vi "ExSpectGetMirrorInfo.vi"() -> ()   [LabVIEW 2010]
panel:
  out "Position":string
  in  "Mirror Number":i16=1 min=1 max=2 step=1
  out "error out":errorcluster
  in  "error in (no error)":errorcluster
  # "ExSpectGetMirrorInfo.vi\n(Normal Spectrograph via USB/COM port)\nThis VI will read the current position of the selected mirror."
  # "1 = Entrance\n 2 = Exit"
  # "NOTES:\nA properly configured spectometer .ini must be present in the LabVIEW folder for spectrograph operation.\n\nConsult the Toolkit documentation for more information on how to configure this file."
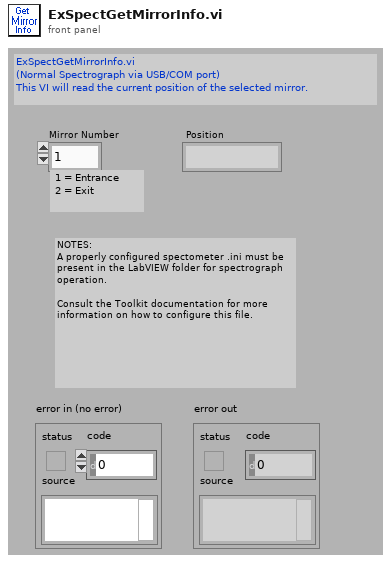
[diagram p1: front panel]
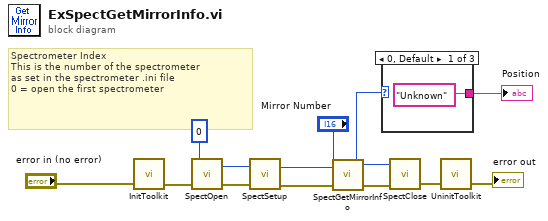
[diagram p0: block diagram]
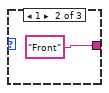
[diagram p2: hidden frame]
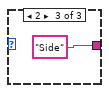
[diagram p3: hidden frame]
diagram:
  # "Spectrometer Index\nThis is the number of the spectrometer\nas set in the spectrometer .ini file\n0 = open the first spectrometer"
  n1 = call <userlib>:"InitToolkit.vi"("error in"="error in (no error)") -> ("error out"=w13:errorcluster)
  n2 = call <userlib>:"SpectOpen.vi"("error in"=w13, "Spectrometer ID"=0) -> ("error out"=w12:errorcluster, "Spectrometer Handle"=w8:u32)  [unwired: 1 in]
  n3 = call <userlib>:"SpectSetup.vi"("error in"=w12, "Spectrometer Handle"=w8) -> ("error out"=w7:errorcluster, "Spectrometer Handle"=w5:u32)
  n4 = call <userlib>:"SpectGetMirrorInfo.vi"("error in"=w7, "Mirror"="Mirror Number", "Spectrometer Handle"=w5) -> ("error out"=w6:errorcluster, "Position"=w2:i16, "Spectrometer Handle"=w3:u32)
  n5 = case shown="0, Default" w2 {
    tunnel: ["Unknown" "Front" "Side"] -> w1
    frame 0, Default {
    }
    frame 1 {
    }
    frame 2 {
    }
  }
  "Position" <- w1
  n6 = call <userlib>:"SpectClose.vi"("error in"=w6, "Spectrometer Handle"=w3) -> ("error out"=w11:errorcluster)
  n7 = call <userlib>:"UninitToolkit.vi"("error in"=w11) -> ("error out"=→"error out":errorcluster)
